vi "Геометрическая последовательность.vi"() -> ()   [LabVIEW 2021]
panel:
  out "Сумма":dbl
  in  "Множитель":dbl
  in  "Первый\nчлен":dbl
  in  "Количество \nЭлеметнов":dbl
  out "Array":dbl[](array[numeric])
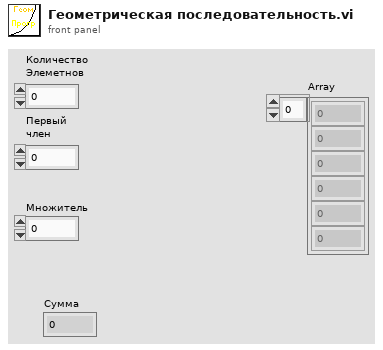
[diagram p1: front panel]
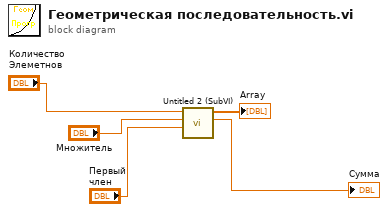
[diagram p0: block diagram]
diagram:
  n1 = call "Untitled 2 (SubVI).vi"("Первый\nчлен"="Первый\nчлен", "Множитель"="Множитель", "Количество \nЭлеметнов"="Количество \nЭлеметнов") -> ("Сумма"=→"Сумма":dbl, "Array"=→"Array":dbl[])  [unwired: 7 in]
